vi "test.StateIterator.vi"() -> ()   [LabVIEW 2017]
uses:
  08aafcae-e060-4efa-a869-0ec527f2211e.vi
  89560828-79ad-4510-8f85-ed9fba072854.vi
  08aafcae-e060-4efa-a869-0ec527f2211e.vi/89031375-ba70-4d5e-9a4b-1a7483d598c0.vi
  JKI/State Iterator.vim/678e7bd1-aa8b-43f7-87bf-d4ddbc903abc.vi
  <userlib>/_OpenG.lib/lvdata/lvdata.llb/Get Strings from Enum__ogtk.vi
panel:
  out "number as enum 2":T1(ring)
  in  "stop":bool
  in  "Boolean":bool
  out "number as enum":T1(ring)
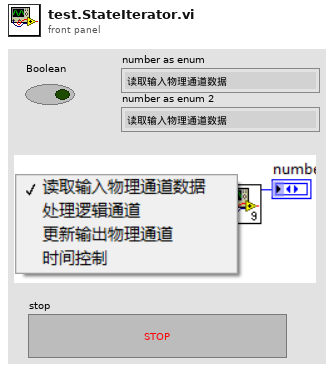
[diagram p1: front panel]
types:
  T1 = enum16{"读取输入物理通道数据", "处理逻辑通道", "更新输出物理通道", "时间控制"}
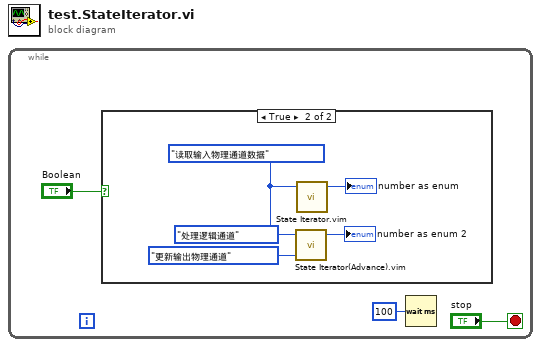
[diagram p0: block diagram]
diagram:
  n1 = while {
    stop <- "stop" stop-if-true
    n2 = case shown="True" "Boolean" {
      frame False {
      }
      frame True {
        w4 = T1."读取输入物理通道数据" ("Enum")
        n3 = call "State Iterator(Advance).vim"("Start State"=T1."处理逻辑通道" ("Enum"), "SM Typedef"=w4, "End State"=T1."更新输出物理通道" ("Enum")) -> ("State"=→"number as enum 2":T1)  [unwired: 4 in]
        n4 = call "State Iterator.vim"("StateMachine Typedef"=w4) -> ("State"=→"number as enum":T1)  [unwired: 6 in]
      }
    }
    n5 = Wait (ms)(milliseconds to wait=u32 100) -> ()  [unwired: 1 out]
  }
